vi "Content.vi"(7 "Context":refnum<class "Context.lvclass">, 8 "Error In":errorcluster, 11 "Section In":refnum<class "Section.lvclass">) -> (0 "Error Out":errorcluster, 2 "Content":string, 3 "Section Out":refnum<class "Section.lvclass">)   [LabVIEW 2018, in "Toolkit.lvlib" / "Nodes.lvlib" / "Section.lvclass"]
uses:
  Section.lvclass
  Data/Context/Context.lvclass
  Section.lvclass/Section.ctl
  Data/Array/Array.lvclass
  Data/Array/Array.lvclass/Array.ctl
  Data/Context/Context.lvclass/Context.ctl
  Data/Boolean/Boolean.lvclass
  Data/Function/Function.lvclass
  Data/String/String.lvclass
  Data/String/String.lvclass/String.ctl
  Data/Abstract/Abstract.lvclass
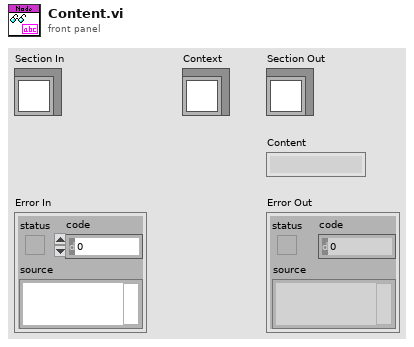
[diagram p1: front panel]
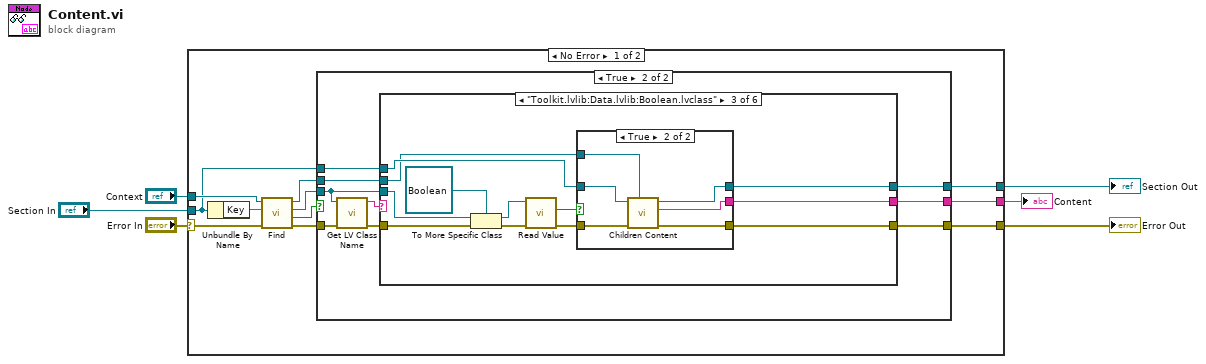
[diagram p0: block diagram]
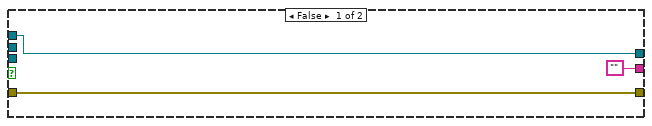
[diagram p2: hidden frame]
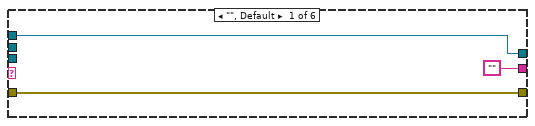
[diagram p3: hidden frame]
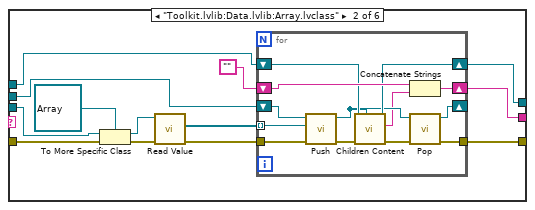
[diagram p4: hidden frame]
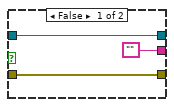
[diagram p5: hidden frame]
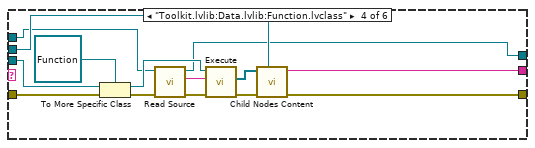
[diagram p6: hidden frame]
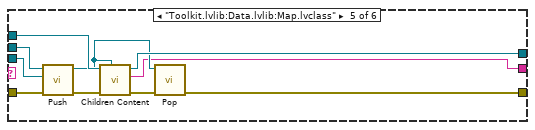
[diagram p7: hidden frame]
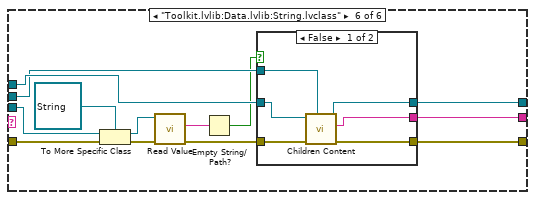
[diagram p8: hidden frame]
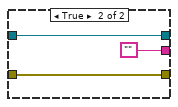
[diagram p9: hidden frame]
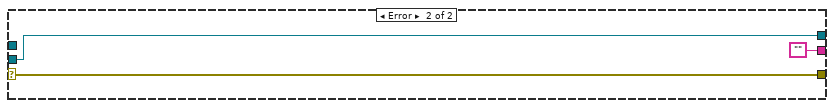
[diagram p10: hidden frame]
diagram:
  n1 = case shown="No Error" "Error In" {
    selector: "Error In" -> [w17 w127]
    tunnel: "Section In" -> [w9 w128]
    tunnel: [w8 w128] -> w4
    tunnel: [w12 w127] -> w3
    tunnel: [w13 ""] -> w2
    tunnel: "Context" -> [w16 _]
    frame No Error {
      n2 = Unbundle By Name(w9) -> ("Key"=w15:string)
      n3 = call "Find.vi"("Error In"=w17, "Key"=w15, "Context In"=w16) -> ("Error Out"=w11:errorcluster, "Found?"=w14:bool, "Datum"=w10:refnum<class "Abstract.lvclass">, "Context Out"=w7:refnum<class "Context.lvclass">)  [unwired: 5 in]
      n4 = case shown="True" w14 {
        tunnel: ["" w26] -> w13
        tunnel: [w19 w25] -> w12
        tunnel: w11 -> [w19 w29]
        tunnel: w10 -> [_ w24]
        tunnel: w9 -> [w18 w23]
        tunnel: [w18 w22] -> w8
        tunnel: w7 -> [_ w21]
        frame False {
        }
        frame True {
          n5 = call <vilib>:"Get LV Class Name.vi"("error in (no error)"=w29, "object"=w24) -> ("error out"=w27:errorcluster, "class name"=w28:string)  [unwired: 8 in]
          n6 = case shown="\"Toolkit.lvlib:Data.lvlib:Boolean.lvclass\"" w28 {
            tunnel: w27 -> [w31 w45 w70 w93 w95 w116]
            tunnel: ["" w35 w63 w86 w94 w114] -> w26
            tunnel: [w31 w37 w62 w87 w102 w113] -> w25
            tunnel: w24 -> [_ w44 w69 w92 w96 w115]
            tunnel: w23 -> [w30 w34 w61 w85 w101 w112]
            tunnel: [w30 w33 w60 w80 w100 w111] -> w22
            tunnel: w21 -> [_ w39 w59 w88 w103 w110]
            frame "", Default {
            }
            frame "Toolkit.lvlib:Data.lvlib:Array.lvclass" {
              n7 = To More Specific Class(target class=refnum<class "Array.lvclass"> refnum ("Toolkit.lvlib:Data.lvlib:Array.lvclass"), reference=w44, error in=w45) -> (specific class reference=w42:refnum<class "Array.lvclass">, error out=w41:errorcluster)
              n8 = call "Read Value.vi"("Error In"=w41, "Array In"=w42) -> ("Error Out"=w38:errorcluster, "Value"=w40:refnum<class "Abstract.lvclass">[])  [unwired: 7 in, 1 out]
              n9 = for {
                tunnel: w40 -> [w56] mode=indexing
                tunnel: w38 -> [w58]
                shift-right: [w55] -> _
                shift-left: w39 -> [w57]
                tunnel: [w54] -> w37
                shift-right: [w52] -> w35
                shift-left: "" -> [w53]
                shift-right: [w50] -> w33
                shift-left: w34 -> [w51]
                n10 = call "Push.vi"("Error In"=w58, "Datum"=w56, "Context In"=w57) -> ("Error Out"=w48:errorcluster, "Context Out"=w49:refnum<class "Context.lvclass">)  [unwired: 7 in]
                n11 = call "Children Content.vi"("Context"=w49, "Error In"=w48, "Section In"=w51) -> ("Error Out"=w47:errorcluster, "Content"=w46:string, "Section Out"=w50:refnum<class "Section.lvclass">)  [unwired: 6 in]
                n12 = Concatenate Strings(w53, w46) -> (w52:string)
                n13 = call "Pop.vi"("Error In"=w47, "Context In"=w49) -> ("Error Out"=w54:errorcluster, "Context Out"=w55:refnum<class "Context.lvclass">)  [unwired: 7 in, 1 out]
              }
            }
            frame "Toolkit.lvlib:Data.lvlib:Boolean.lvclass" {
              n14 = To More Specific Class(target class=refnum<class "Boolean.lvclass"> refnum ("Toolkit.lvlib:Data.lvlib:Boolean.lvclass"), reference=w69, error in=w70) -> (specific class reference=w66:refnum<class "Boolean.lvclass">, error out=w67:errorcluster)
              n15 = call "Read Value.vi"("Error In"=w67, "Boolean In"=w66) -> ("Error Out"=w64:errorcluster, "Value"=w65:bool)  [unwired: 7 in, 1 out]
              n16 = case shown="True" w65 {
                tunnel: w64 -> [w72 w79]
                tunnel: ["" w75] -> w63
                tunnel: [w72 w76] -> w62
                tunnel: w61 -> [w71 w78]
                tunnel: [w71 w77] -> w60
                tunnel: w59 -> [_ w74]
                frame False {
                }
                frame True {
                  n17 = call "Children Content.vi"("Context"=w74, "Error In"=w79, "Section In"=w78) -> ("Error Out"=w76:errorcluster, "Content"=w75:string, "Section Out"=w77:refnum<class "Section.lvclass">)  [unwired: 6 in]
                }
              }
            }
            frame "Toolkit.lvlib:Data.lvlib:Function.lvclass" {
              n18 = To More Specific Class(target class=refnum<class "Function.lvclass"> refnum ("Toolkit.lvlib:Data.lvlib:Function.lvclass"), reference=w92, error in=w93) -> (specific class reference=w90:refnum<class "Function.lvclass">, error out=w83:errorcluster)
              n19 = call "Read Source.vi"("Error In"=w83, "Section In"=w85) -> ("Error Out"=w82:errorcluster, "Source"=w81:string, "Section Out"=w80:refnum<class "Section.lvclass">)  [unwired: 7 in]
              n20 = call-dynamic "Execute.vi"("Error In"=w82, "Source"=w81, "Function In"=w90) -> ("Error Out"=w84:errorcluster, "Nodes"=w89:refnum<class "Abstract.lvclass">[])  [unwired: 6 in, 1 out]
              n21 = call "Child Nodes Content.vi"("Context"=w88, "Error In"=w84, "Children"=w89) -> ("Error Out"=w87:errorcluster, "Content"=w86:string)  [unwired: 7 in]
            }
            frame "Toolkit.lvlib:Data.lvlib:Map.lvclass" {
              n22 = call "Push.vi"("Error In"=w95, "Datum"=w96, "Context In"=w103) -> ("Error Out"=w98:errorcluster, "Context Out"=w99:refnum<class "Context.lvclass">)  [unwired: 7 in]
              n23 = call "Children Content.vi"("Context"=w99, "Error In"=w98, "Section In"=w101) -> ("Error Out"=w97:errorcluster, "Content"=w94:string, "Section Out"=w100:refnum<class "Section.lvclass">)  [unwired: 6 in]
              n24 = call "Pop.vi"("Error In"=w97, "Context In"=w99) -> ("Error Out"=w102:errorcluster)  [unwired: 7 in, 2 out]
            }
            frame "Toolkit.lvlib:Data.lvlib:String.lvclass" {
              n25 = To More Specific Class(target class=refnum<class "String.lvclass"> refnum ("Toolkit.lvlib:Data.lvlib:String.lvclass"), reference=w115, error in=w116) -> (specific class reference=w107:refnum<class "String.lvclass">, error out=w108:errorcluster)
              n26 = call "Read Value.vi"("Error In"=w108, "String In"=w107) -> ("Error Out"=w104:errorcluster, "Value"=w106:string)  [unwired: 7 in, 1 out]
              n27 = Empty String/Path?(string/path=w106) -> (empty?=w105:bool)
              n28 = case shown="False" w105 {
                tunnel: [w119 ""] -> w114
                tunnel: [w120 w123] -> w113
                tunnel: w112 -> [w122 w124]
                tunnel: [w121 w124] -> w111
                tunnel: w110 -> [w117 _]
                tunnel: w104 -> [w118 w123]
                frame False {
                  n29 = call "Children Content.vi"("Context"=w117, "Error In"=w118, "Section In"=w122) -> ("Error Out"=w120:errorcluster, "Content"=w119:string, "Section Out"=w121:refnum<class "Section.lvclass">)  [unwired: 6 in]
                }
                frame True {
                }
              }
            }
          }
        }
      }
    }
    frame Error {
    }
  }
  "Error Out" <- w3
  "Section Out" <- w4
  "Content" <- w2
